vi "AlazarGetSDKVersion.vi"(11 "error in (no error)":errorcluster) -> (4 "Major Number":u8, 6 "Minor Number":u8, 8 "Revision Number":u8, 10 "Return Code":u32, 15 "error out":errorcluster)   [LabVIEW 2009]
doc: "Get the driver library version. This is the version of ATSApi.dll under Windows, or ATSApi.so under Linux."
uses:
  ATSApi.dll
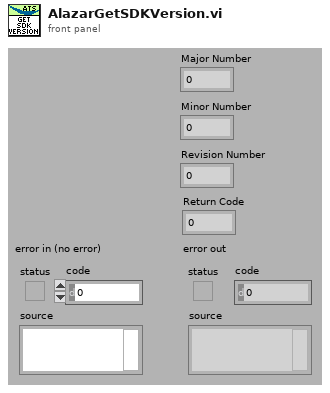
[diagram p1: front panel]
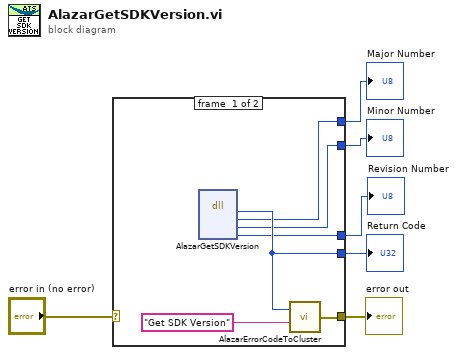
[diagram p0: block diagram]
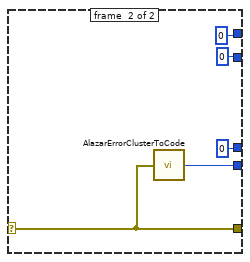
[diagram p2: hidden frame]
diagram:
  n1 = case shown="No Error" "error in (no error)" {
    selector: "error in (no error)" -> [_ w17]
    tunnel: [w10 w17] -> w5
    tunnel: [w12 w16] -> w4
    tunnel: [w9 0] -> w3
    tunnel: [w8 0] -> w2
    tunnel: [w7 0] -> w1
    frame #0 {
      n2 = dll-call lib="ATSApi.dll" fn="AlazarGetSDKVersion"() -> (w12:u32, "majorVersion"=w9:u8, "minorVersion"=w8:u8, "revisionNumber"=w7:u8)  [unwired: 6 in, 2 out]
      n3 = call "AlazarErrorCodeToCluster.vi"("Message"="Get SDK Version", "Error Code"=w12) -> ("error out"=w10:errorcluster)
    }
    frame #1 {
      n4 = call "AlazarErrorClusterToCode.vi"("error in (no error)"=w17) -> ("Error Code"=w16:u32)
    }
  }
  "error out" <- w5
  "Return Code" <- w4
  "Major Number" <- w3
  "Minor Number" <- w2
  "Revision Number" <- w1
